vi "Write Boolean Colors Props.vi"(8 "error in (no error)":errorcluster, 10 "Boolean Colors Props":T1, 11 "Control in":refnum<vi>) -> (0 "error out":errorcluster, 3 "Control":refnum<vi>)   [LabVIEW 2020, in "VolatusGUIEditorCore.lvlib"]
uses:
  VolatusGUIEditorCore.lvlib
  Boolean Color Props.ctl
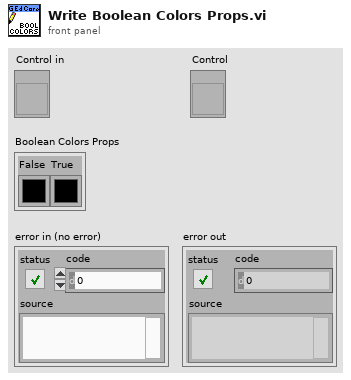
[diagram p1: front panel]
types:
  T1 = typedef "VolatusGUIEditorCore.lvlib/Boolean Color Props.ctl" = cluster{"False":u32, "True":u32}
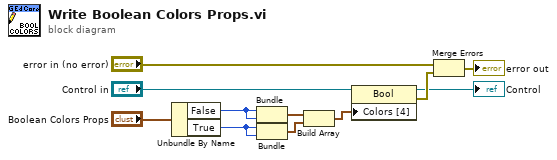
[diagram p0: block diagram]
diagram:
  n1 = Unbundle By Name("Boolean Colors Props") -> ("False"=w8:u32, "True"=w7:u32)
  n2 = Bundle("False"=w8, "False"=w8) -> (w6:cluster{"False":u32, "False":u32})  [unwired: 1 in]
  n3 = Bundle("True"=w7, "True"=w7) -> (w5:cluster{"True":u32, "True":u32})  [unwired: 1 in]
  n4 = Build Array(w6, w5) -> (w4:cluster{"True":u32, "True":u32}[])
  n5 = property class="Bool"(reference="Control in", "Colors [4]"=w4) -> (reference out=→"Control":refnum<vi>, error out=w11:errorcluster)  [unwired: 1 in]
  n6 = Merge Errors("error in (no error)", w11) -> (→"error out":errorcluster)
